vi "From JSON Tree.vi"(8 "error in (no error)":errorcluster, 10 "JSON in":refnum<class "JSON Datatype.lvclass">, 11 "Response in":refnum<class "Response.lvclass">) -> (0 "error out":errorcluster, 3 "Response out":refnum<class "Response.lvclass">)   [LabVIEW 2015, in "Response.lvclass"]
uses:
  Response.lvclass
  <vilib>/National Instruments/JSON Support for LabVIEW/JSON Data Classes/JSON Datatype/JSON Datatype.lvclass
  id/id.lvclass
  New folder/result.lvclass
  error/error.lvclass
  Response.lvclass/Response.ctl
  <vilib>/National Instruments/JSON Support for LabVIEW/JSON Data Classes/JSON Datatype/To More Specific Type (Object).vi
  <vilib>/National Instruments/JSON Support for LabVIEW/JSON Data Classes/JSON Object/Get Value (String Value).vi
  <vilib>/National Instruments/JSON Support for LabVIEW/JSON Data Classes/JSON Object/Get Value (JSON).vi
  <vilib>/National Instruments/JSON Support for LabVIEW/JSON Data Classes/JSON Object/Get Value (Object).vi
  <vilib>/National Instruments/JSON Support for LabVIEW/JSON Data Classes/JSON Object/JSON Object.lvclass
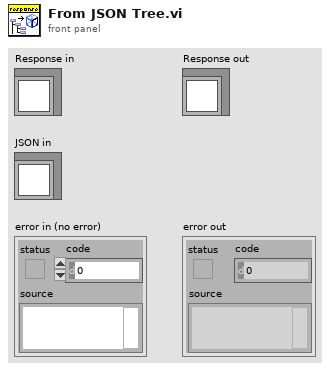
[diagram p1: front panel]
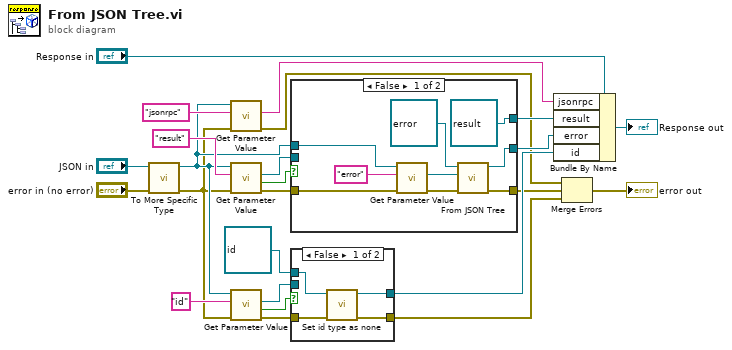
[diagram p0: block diagram]
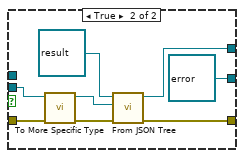
[diagram p2: hidden frame]
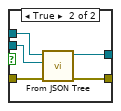
[diagram p3: hidden frame]
diagram:
  n1 = call-poly <vilib>:"To More Specific Type.vi"("error in (no error)"="error in (no error)", "JSON Datatype in"="JSON in") -> ("error out"=w3:errorcluster, "JSON Datatype out"=w5:refnum<class "JSON Object.lvclass">)  [unwired: 8 in]
  n2 = call-poly <vilib>:"Get Parameter Value.vi"("error in (no error)"=w3, "key"="jsonrpc" ("Parameter Name"), "JSON Object in"=w5) -> ("error out"=w10:errorcluster, "value"=w1:string)  [unwired: 6 in, 1 out]
  n3 = call-poly <vilib>:"Get Parameter Value.vi"("error in (no error)"=w3, "key"="result" ("Parameter Name"), "JSON Object in"=w5) -> ("error out"=w8:errorcluster, "found"=w16:bool, "value"=w15:refnum<class "JSON Datatype.lvclass">)  [unwired: 6 in]
  n4 = call-poly <vilib>:"Get Parameter Value.vi"("error in (no error)"=w3, "key"="id" ("Parameter Name"), "JSON Object in"=w5) -> ("error out"=w11:errorcluster, "found"=w12:bool, "value"=w2:refnum<class "JSON Object.lvclass">)  [unwired: 6 in]
  n5 = case shown="False" w16 {
    tunnel: w15 -> [_ w38]
    tunnel: [refnum<class "result.lvclass"> refnum ("result out") w41] -> w14
    tunnel: [w30 refnum<class "error.lvclass"> refnum ("error")] -> w13
    tunnel: w5 -> [w32 _]
    tunnel: [w26 w36] -> w9
    tunnel: w8 -> [w28 w34]
    frame False {
      n6 = call-poly <vilib>:"Get Parameter Value.vi"("error in (no error)"=w28, "key"="error", "JSON Object in"=w32) -> ("error out"=w27:errorcluster, "value"=w25:refnum<class "JSON Object.lvclass">)  [unwired: 6 in, 1 out]
      n7 = call-dynamic "From JSON Tree.vi"("error in (no error)"=w27, "JSON in"=w25, "error in"=refnum<class "error.lvclass"> refnum) -> (0:"error out"=w26:errorcluster, 3:"error out"=w30:refnum<class "error.lvclass">)  [unwired: 7 in]
    }
    frame True {
      n8 = call-poly <vilib>:"To More Specific Type.vi"("error in (no error)"=w34, "JSON Datatype in"=w38) -> ("error out"=w35:errorcluster, "JSON Datatype out"=w37:refnum<class "JSON Object.lvclass">)  [unwired: 8 in]
      n9 = call-dynamic "From JSON Tree.vi"("error in (no error)"=w35, "JSON in"=w37, "result in"=refnum<class "result.lvclass"> refnum) -> ("error out"=w36:errorcluster, "result out"=w41:refnum<class "result.lvclass">)  [unwired: 7 in]
    }
  }
  n10 = case shown="False" w12 {
    tunnel: refnum<class "id.lvclass"> refnum ("id.lvclass") -> [w45 w50]
    tunnel: [w44 w49] -> w20
    tunnel: [w43 w48] -> w7
    tunnel: w2 -> [_ w47]
    tunnel: w11 -> [w42 w46]
    frame False {
      n11 = call-dynamic "Set id type as none.vi"("error in (no error)"=w42, "id in"=w45) -> ("error out"=w43:errorcluster, "id out"=w44:refnum<class "id.lvclass">)  [unwired: 8 in]
    }
    frame True {
      n12 = call-dynamic "From JSON Tree.vi"("error in (no error)"=w46, "JSON in"=w47, "id in"=w50) -> ("error out"=w48:errorcluster, "id out"=w49:refnum<class "id.lvclass">)  [unwired: 7 in]
    }
  }
  n13 = Bundle By Name(cluster="Response in", "jsonrpc"=w1, "result"=w14, "error"=w13, "id"=w20) -> (→"Response out":refnum<class "Response.lvclass">)
  n14 = Merge Errors(w10, w9, w7) -> (→"error out":errorcluster)
